vi "queue sm 0.vi"() -> ()   [LabVIEW 2020]
uses:
  file I O/ASSIGN 8/que sm states.ctl
panel:
  out "State output":string
  out "state":T1
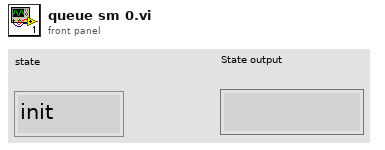
[diagram p1: front panel]
types:
  T1 = typedef "que sm states.ctl" = enum16{"init", "events", "state 1", "state 2", "stop"}
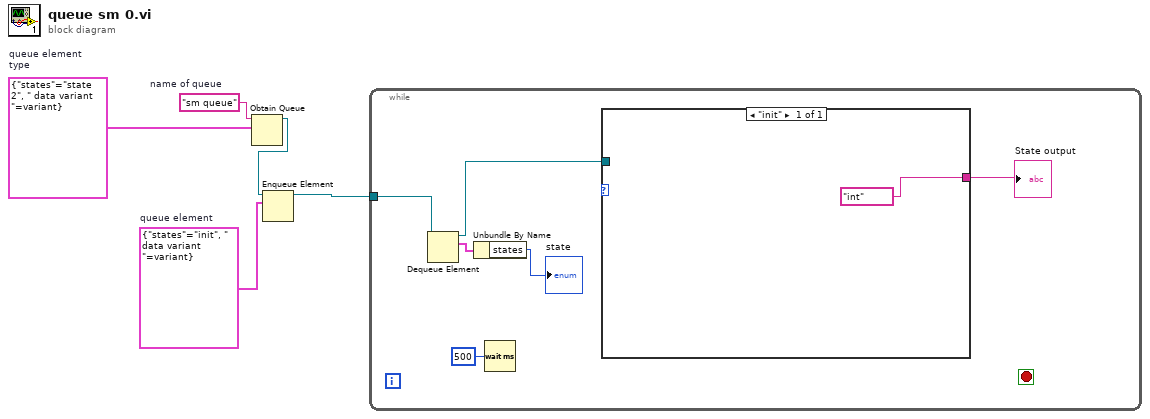
[diagram p0: block diagram]
diagram:
  w1 = cluster{"states":T1, " data variant ":variant} {"states"=enum."init", " data variant "=variant(i32[][] [[0, 0, 0], [0, 0, 0]])}  # queue element
  w2 = cluster{"states":T1, " data variant ":variant} {"states"=enum."state 2", " data variant "=variant(i32[][] [[0, 0, 0], [0, 0, 0]])}  # queue element type
  w5 = "sm queue"  # name of queue
  n1 = Obtain Queue(name (unnamed)=w5, element data type=w2) -> (queue out=w4:refnum<queue>)  [unwired: 3 in, 2 out]
  n2 = Enqueue Element(queue=w4, element=w1) -> (queue out=w3:refnum<queue>)  [unwired: 2 in, 2 out]
  n3 = while {
    tunnel: w3 -> [w9]
    stop <- _ stop-if-true
    n4 = Dequeue Element(queue=w9) -> (queue out=w8:refnum<queue>, element=w11:cluster{"states":T1, " data variant ":variant})  [unwired: 2 in, 2 out]
    n5 = Unbundle By Name(w11) -> ("states"=→"state":T1)
    n6 = Wait (ms)(milliseconds to wait=u32 500) -> ()  [unwired: 1 out]
    n7 = case shown="\"init\"" {
      selector: _ -> [_]
      tunnel: w8 -> [_]
      tunnel: ["int"] -> w6
      frame "init" {
      }
    }
    "State output" <- w6
  }
